vi "Write Child Attributes.vi"(10 "Child Attributes":T1, 11 "Base Actor in":refnum<class "Base Actor.lvclass">) -> (3 "Base Actor out":refnum<class "Base Actor.lvclass">)   [LabVIEW 2020, in "jettl.lvlib" / "Base jettl Actor.lvlib" / "Base Actor.lvlib" / "Base Actor.lvclass"]
uses:
  Base Actor.lvclass
  Msg/Msg.lvclass
  Actor/Actor.lvclass
  Transport/Transport.lvclass
  Attributes Metadata/Attributes Metadata.lvclass
  Base Actor.lvclass/Base Actor.ctl
  Child Attributes.ctl
  jettl.lvlib
  Msgs.ctl
  Attributes.ctl
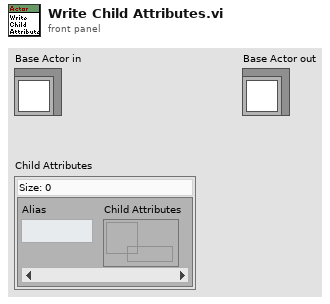
[diagram p1: front panel]
types:
  T1 = typedef "jettl.lvlib/Child Attributes.ctl" = map{string, refnum<data-value>}
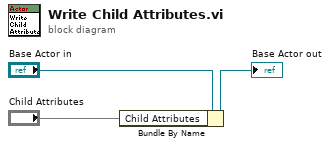
[diagram p0: block diagram]
diagram:
  n1 = Bundle By Name(cluster="Base Actor in", "Child Attributes"="Child Attributes") -> (→"Base Actor out":refnum<class "Base Actor.lvclass">)
